vi "Configure Output Timer.vi"(6 "Enable Output Timer (T: Enable)":bool=TRUE, 8 "error in (no error)":errorcluster, 9 "Enable Output (T: Enable)":bool=TRUE, 10 "Output Timer(0)":dbl format="%#_2g", 11 "VISA resource name":refnum<visa-resource-name>) -> (0 "error out":errorcluster, 3 "VISA resource name out":refnum<visa-resource-name>)   [LabVIEW 2021, in "Keithley 2200 Series.lvlib"]
doc: "Configure the output-timer. \nTo start Timer \n- First, set OUTPUT:TIMER ON, then set OUTPUT ON. \nTo end Timer \n- Set OUTPUT:TIMER OFF to turn timer off."
uses:
  <instrlib>/Keithley 2200 Series/Keithley 2200 Series.lvlib
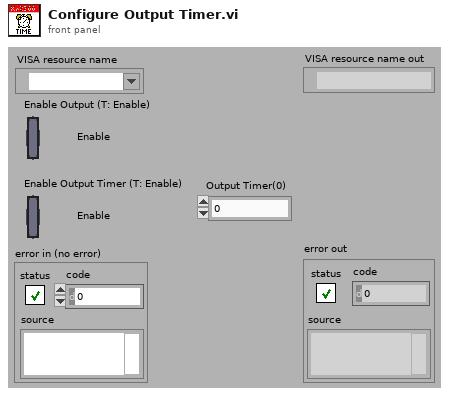
[diagram p1: front panel]
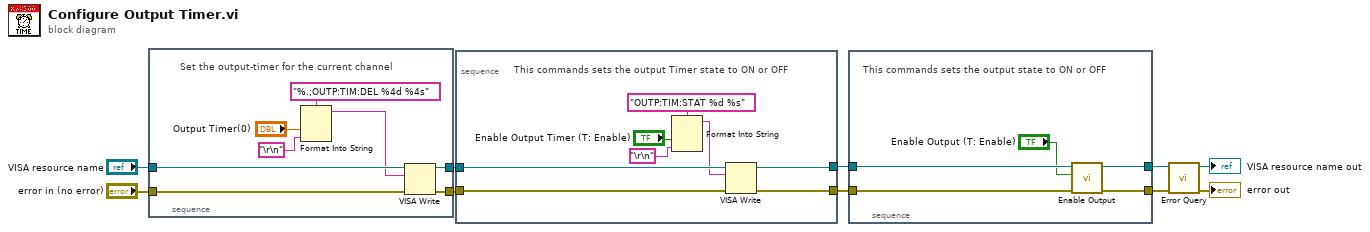
[diagram p0: block diagram]
diagram:
  n1 = stacked-sequence {
    tunnel: "VISA resource name" -> [w18]
    tunnel: "error in (no error)" -> [w17]
    tunnel: [w12] -> w6
    tunnel: [w11] -> w5
    frame #0 {
      # "Set the output-timer for the current channel"
      n2 = Format Into String(format string="%.;OUTP:TIM:DEL %4d %4s", "Output Timer(0)", "\r\n") -> (resulting string=w14:string)  [unwired: 2 in, 1 out]
      n3 = VISA Write(VISA resource name=w18, write buffer=w14, error in (no error)=w17) -> (VISA resource name out=w12:refnum<visa-resource-name>, error out=w11:errorcluster)  [unwired: 1 out]
    }
  }
  n4 = stacked-sequence {
    tunnel: w6 -> [w24]
    tunnel: w5 -> [w23]
    tunnel: [w22] -> w4
    tunnel: [w21] -> w3
    frame #0 {
      # "This commands sets the output Timer state to ON or OFF"
      n5 = Format Into String(format string="OUTP:TIM:STAT %d %s", "Enable Output Timer (T: Enable)", "\r\n") -> (resulting string=w20:string)  [unwired: 2 in, 1 out]
      n6 = VISA Write(VISA resource name=w24, write buffer=w20, error in (no error)=w23) -> (VISA resource name out=w22:refnum<visa-resource-name>, error out=w21:errorcluster)  [unwired: 1 out]
    }
  }
  n7 = stacked-sequence {
    tunnel: w4 -> [w31]
    tunnel: w3 -> [w30]
    tunnel: [w29] -> w2
    tunnel: [w28] -> w1
    frame #0 {
      # "This commands sets the output state to ON or OFF"
      n8 = call <instrlib>:"Enable Output.vi"("error in (no error)"=w30, "Enable Output (T: Enable)"="Enable Output (T: Enable)", "VISA resource name"=w31) -> ("error out"=w28:errorcluster, "VISA resource name out"=w29:refnum<visa-resource-name>)  [unwired: 7 out]
    }
  }
  n9 = call <instrlib>:"Error Query.vi"("error in (no error)"=w1, "VISA resource name"=w2) -> ("error out"=→"error out":errorcluster, "VISA resource name out"=→"VISA resource name out":refnum<visa-resource-name>)  [unwired: 8 out]
